vi "PROYECTOICEUWU.vi"(7 "DI Channel":u8, 8 "error in (no error)":errorcluster, 9 "LINX Resource in":T1, 10 "DO Channel 2":u8, 11 "DO Channel":u8) -> (0 "error out":errorcluster, 1 "10":bool, 2 "Boolean":bool, 3 "11":bool, 4 "01":bool, 5 "LINX Resource out":T1, 6 "00":bool)   [LabVIEW 2026]
uses:
  <vilib>/MakerHub/LINX/LMH-LINX.lvlib
  <vilib>/MakerHub/LINX/Public/Peripherals/Digital/Digital Write 1 Chan.vi
  <vilib>/MakerHub/LINX/Public/Peripherals/Digital/Digital Read 1 Chan.vi
  <vilib>/MakerHub/LINX/Private/Type Defs/Platform.ctl
  <vilib>/MakerHub/LINX/Private/Type Defs/Interface.ctl
  <vilib>/MakerHub/LINX/Private/Device/Type Defs/TCP Config.ctl
  <vilib>/MakerHub/LINX/Private/Device/Device.lvlib
  <vilib>/MakerHub/LINX/Private/Device/Type Defs/Channels.ctl
  <vilib>/MakerHub/LINX/Private/Device/Type Defs/LINX Device Config.ctl
  <vilib>/MakerHub/LINX/Private/Type Defs/LINX Ref.ctl
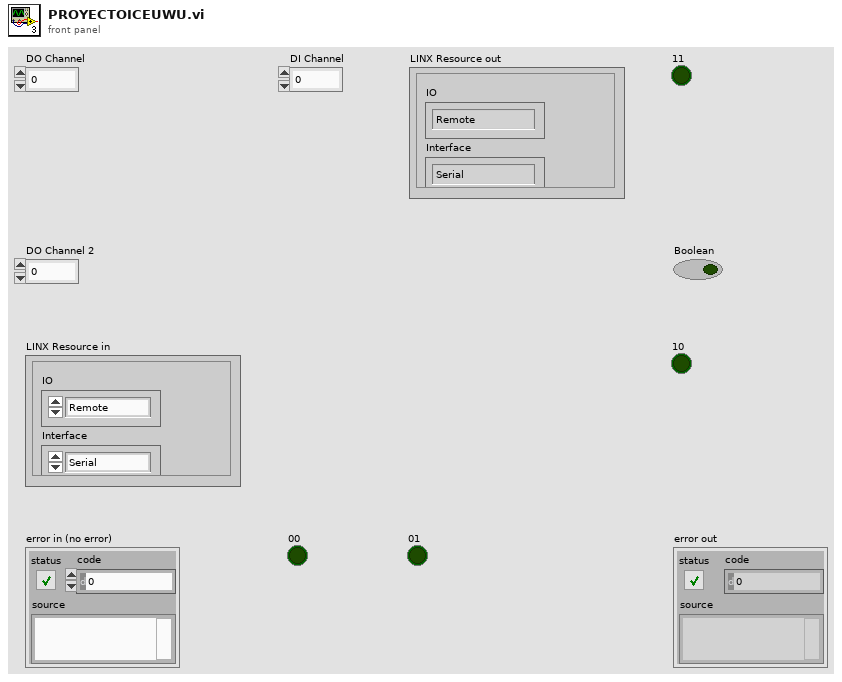
[diagram p1: front panel]
types:
  T1 = typedef "LMH-LINX.lvlib/LINX Ref.ctl" = cluster{"IO":T2, "Interface":T3, "LINX Device Config":T4}
  T2 = typedef "LMH-LINX.lvlib/Platform.ctl" = enum16{"Remote", "Local"}
  T3 = typedef "LMH-LINX.lvlib/Interface.ctl" = enum16{"Serial", "TCP"}
  T4 = typedef "LMH-LINX.lvlib/Device.lvlib/LINX Device Config.ctl" = cluster{"Interface":T3, "COM Port":refnum<visa-resource-name>, "TCP Configuration":T5, "Device Family":u8, "Device ID":u8, "Device Name":string, "TCP Ref":refnum<k5>, "Channels":T6}
  T5 = typedef "LMH-LINX.lvlib/Device.lvlib/TCP Config.ctl" = cluster{"IP Address":string, "Port":u16}
  T6 = typedef "LMH-LINX.lvlib/Channels.ctl" = cluster{"DI":u8[], "DO":u8[], "AI":u8[], "AO":u8[], "PWM":u8[], "QE":u8[], "UART":u8[], "I2C 2":u8[], "SPI":u8[], "CAN":u8[], "Servo":u8[], "AI Ref (V)":dbl, "AI Resolution (Bits)":u8, "AO Ref (V)":dbl, "AO Resolution (Bits)":u8}
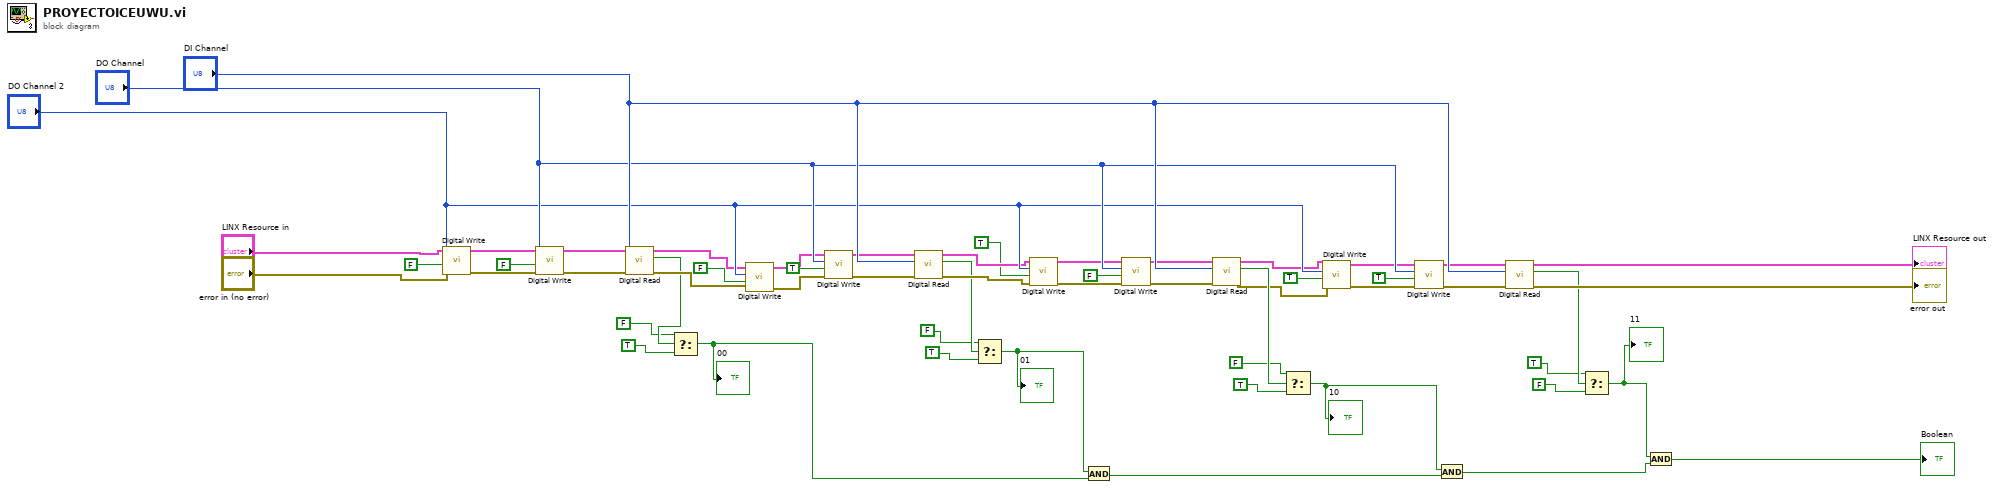
[diagram p0: block diagram]
diagram:
  n1 = call-poly <vilib>:"Digital Write.vi"("Error In"="error in (no error)", "Output Value"=FALSE, "DO Channel"="DO Channel 2", "LINX Resource"="LINX Resource in") -> ("Error Out"=w2:errorcluster, "LINX Resource"=w1:T1)  [unwired: 6 in]
  n2 = call-poly <vilib>:"Digital Write.vi"("Error In"=w2, "Output Value"=FALSE, "DO Channel"="DO Channel", "LINX Resource"=w1) -> ("Error Out"=w4:errorcluster, "LINX Resource"=w3:T1)  [unwired: 6 in]
  n3 = call-poly <vilib>:"Digital Read.vi"("Error In"=w4, "DI Channel"="DI Channel", "LINX Resource"=w3) -> ("Error Out"=w19:errorcluster, "DI Value"=w11:bool, "LINX Resource"=w18:T1)  [unwired: 6 in]
  n4 = Select(t=FALSE, s=w11, f=TRUE ("y")) -> (s? t:f=w48:bool)
  "00" <- w48
  n5 = call-poly <vilib>:"Digital Write.vi"("Error In"=w19, "Output Value"=FALSE, "DO Channel"="DO Channel 2", "LINX Resource"=w18) -> ("Error Out"=w13:errorcluster, "LINX Resource"=w12:T1)  [unwired: 6 in]
  n6 = call-poly <vilib>:"Digital Write.vi"("Error In"=w13, "Output Value"=TRUE, "DO Channel"="DO Channel", "LINX Resource"=w12) -> ("Error Out"=w15:errorcluster, "LINX Resource"=w14:T1)  [unwired: 6 in]
  n7 = call-poly <vilib>:"Digital Read.vi"("Error In"=w15, "DI Channel"="DI Channel", "LINX Resource"=w14) -> ("Error Out"=w36:errorcluster, "DI Value"=w22:bool, "LINX Resource"=w35:T1)  [unwired: 6 in]
  n8 = Select(t=FALSE, s=w22, f=TRUE ("y")) -> (s? t:f=w47:bool)
  "01" <- w47
  n9 = call-poly <vilib>:"Digital Write.vi"("Error In"=w36, "Output Value"=TRUE, "DO Channel"="DO Channel 2", "LINX Resource"=w35) -> ("Error Out"=w24:errorcluster, "LINX Resource"=w23:T1)  [unwired: 6 in]
  n10 = And(x=w47, y=w48) -> (x .and. y?=w50:bool)
  n11 = call-poly <vilib>:"Digital Write.vi"("Error In"=w24, "Output Value"=FALSE, "DO Channel"="DO Channel", "LINX Resource"=w23) -> ("Error Out"=w26:errorcluster, "LINX Resource"=w25:T1)  [unwired: 6 in]
  n12 = call-poly <vilib>:"Digital Read.vi"("Error In"=w26, "DI Channel"="DI Channel", "LINX Resource"=w25) -> ("Error Out"=w38:errorcluster, "DI Value"=w41:bool, "LINX Resource"=w37:T1)  [unwired: 6 in]
  n13 = Select(t=FALSE, s=w41, f=TRUE ("y")) -> (s? t:f=w49:bool)
  "10" <- w49
  n14 = call-poly <vilib>:"Digital Write.vi"("Error In"=w38, "Output Value"=TRUE, "DO Channel"="DO Channel 2", "LINX Resource"=w37) -> ("Error Out"=w30:errorcluster, "LINX Resource"=w29:T1)  [unwired: 6 in]
  n15 = call-poly <vilib>:"Digital Write.vi"("Error In"=w30, "Output Value"=TRUE, "DO Channel"="DO Channel", "LINX Resource"=w29) -> ("Error Out"=w32:errorcluster, "LINX Resource"=w31:T1)  [unwired: 6 in]
  n16 = And(x=w49, y=w50) -> (x .and. y?=w52:bool)
  n17 = call-poly <vilib>:"Digital Read.vi"("Error In"=w32, "DI Channel"="DI Channel", "LINX Resource"=w31) -> ("Error Out"=→"error out":errorcluster, "DI Value"=w44:bool, "LINX Resource"=→"LINX Resource out":T1)  [unwired: 6 in]
  n18 = Select(t=TRUE, s=w44, f=FALSE ("y")) -> (s? t:f=w51:bool)
  "11" <- w51
  n19 = And(x=w51, y=w52) -> (x .and. y?=→"Boolean":bool)
